vi "PPL Version Pre-Build Action.vi"(6 "Top Level/Always Included VIs":path[](array[path]), 7 "Main Destination Path":path, 9 "Target Name":string, 10 "Build Specification Name":string, 11 "Project Path":path) -> (0 "error out":errorcluster)   [LabVIEW 2023]
panel:
  in  "error in (no error)":errorcluster
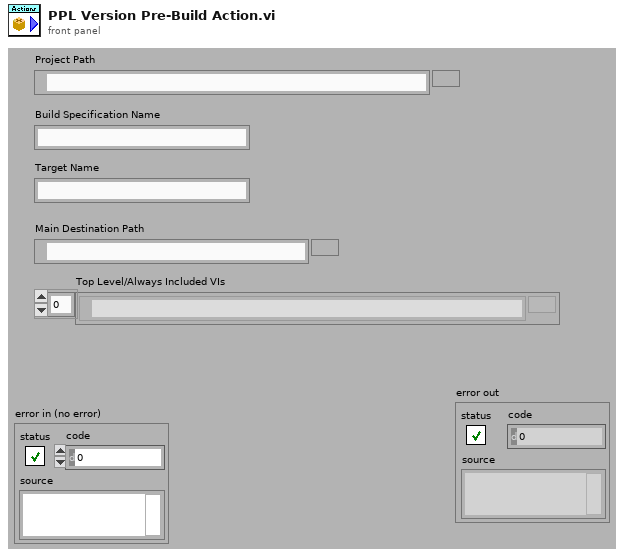
[diagram p1: front panel]
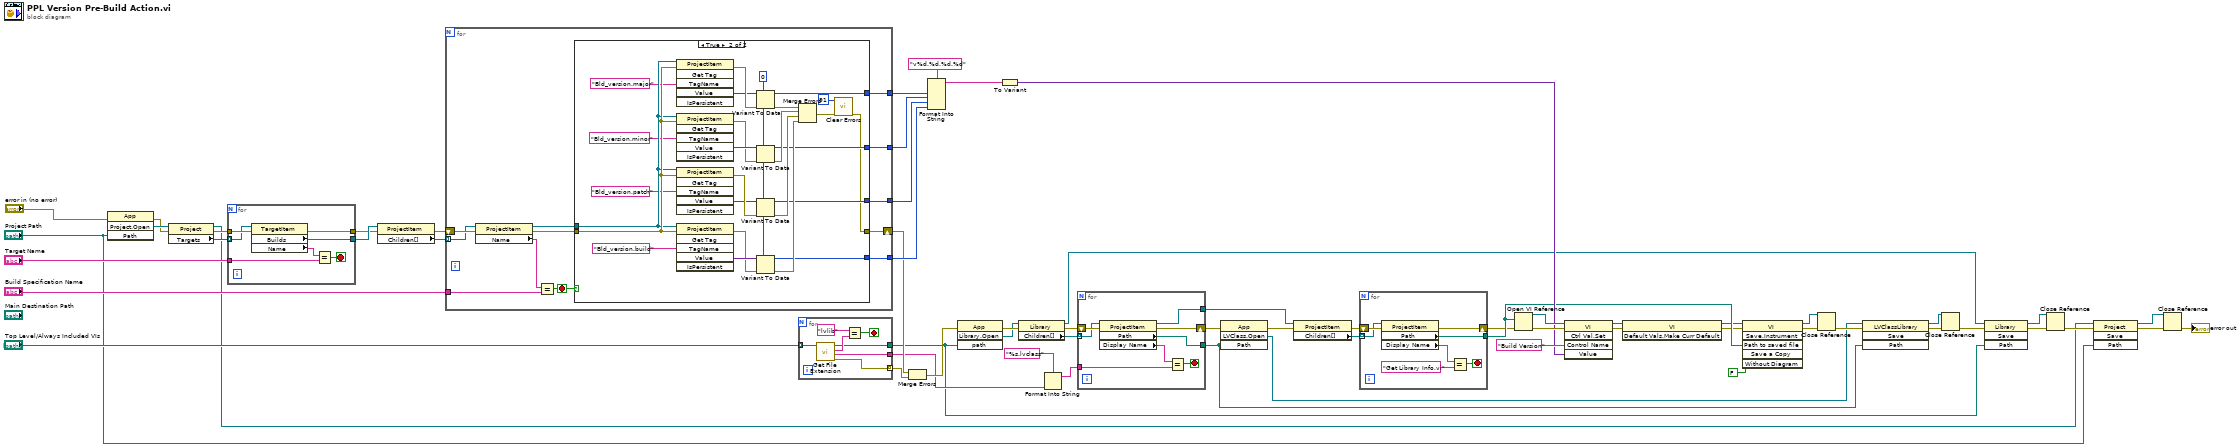
[diagram p0: block diagram]
diagram:
  n1 = invoke class="App" method="Project.Open"(error in="error in (no error)", "Path"="Project Path") -> (error out=w59:errorcluster, "Project:Open"=w62:refnum<vi>)  [unwired: 2 in, 2 out]
  n2 = property class="Project"(reference=w62, error in=w59) -> (reference out=w14:refnum<vi>, error out=w58:errorcluster, "Targets"=w60:refnum<vi>[])
  n3 = for {
    tunnel: w60 -> [w68] mode=indexing
    tunnel: w58 -> [w69]
    tunnel: "Target Name" -> [w67]
    tunnel: [w65] -> w56
    tunnel: [w63] -> w57
    stop <- w66 stop-if-true
    n4 = property class="TargetItem"(reference=w68, error in=w69) -> (error out=w65:errorcluster, "Builds"=w63:refnum<vi>, "Name"=w64:string)  [unwired: 1 out]
    n5 = Equal?(x=w64, y=w67) -> (x = y?=w66:bool)
  }
  n6 = property class="ProjectItem"(reference=w57, error in=w56) -> (error out=w55:errorcluster, "Children[]"=w54:refnum<vi>[])  [unwired: 1 out]
  n7 = for {
    tunnel: "Build Specification Name" -> [w80]
    shift-right: [w79] -> w45
    shift-left: w55 -> [w78]
    tunnel: w54 -> [w77] mode=indexing
    tunnel: [w74] -> w52
    tunnel: [w72] -> w51
    tunnel: [w71] -> w50
    tunnel: [w70] -> w49
    stop <- w73 stop-if-true
    n8 = property class="ProjectItem"(reference=w77) -> (reference out=w75:refnum<vi>, "Name"=w76:string)  [unwired: 1 in, 1 out]
    n9 = Equal?(x=w76, y=w80) -> (x = y?=w73:bool)
    n10 = case shown="True" w73 {
      tunnel: w78 -> [w81 w107]
      tunnel: w75 -> [_ w106]
      tunnel: [w81 w83] -> w79
      tunnel: [_ w89] -> w74
      tunnel: [_ w88] -> w72
      tunnel: [_ w87] -> w71
      tunnel: [_ w86] -> w70
      frame False {
      }
      frame True {
        w93 = u32 0
        n11 = invoke class="ProjectItem" method="Get Tag"(reference=w106, error in=w107, "TagName"="Bld_version.major") -> (error out=w101:errorcluster, "Value"=w100:variant)  [unwired: 3 in, 4 out]
        n12 = invoke class="ProjectItem" method="Get Tag"(reference=w106, error in=w107, "TagName"="Bld_version.minor") -> (error out=w98:errorcluster, "Value"=w99:variant)  [unwired: 3 in, 4 out]
        n13 = invoke class="ProjectItem" method="Get Tag"(reference=w106, error in=w107, "TagName"="Bld_version.patch") -> (error out=w95:errorcluster, "Value"=w94:variant)  [unwired: 3 in, 4 out]
        n14 = invoke class="ProjectItem" method="Get Tag"(reference=w106, error in=w107, "TagName"="Bld_version.build") -> (error out=w96:errorcluster, "Value"=w97:variant)  [unwired: 3 in, 4 out]
        n15 = Variant To Data(error in=w101, type=w93, Variant=w100) -> (data=w89:u32, error out=w85:errorcluster)
        n16 = Variant To Data(error in=w98, type=w93, Variant=w99) -> (data=w88:u32, error out=w92:errorcluster)
        n17 = Variant To Data(error in=w95, type=w93, Variant=w94) -> (data=w87:u32, error out=w91:errorcluster)
        n18 = Variant To Data(error in=w96, type=w93, Variant=w97) -> (data=w86:u32, error out=w90:errorcluster)
        n19 = Merge Errors(w85, w92, w91, w90) -> (w84:errorcluster)
        n20 = call <vilib>:"Clear Errors.vi"("error in (no error)"=w84, "specific error code to clear (0: all)"=91) -> ("error out"=w83:errorcluster)  [unwired: 4 in, 1 out]
      }
    }
  }
  n21 = for {
    tunnel: "Top Level/Always Included VIs" -> [w114] mode=indexing
    tunnel: [w110] -> w18
    tunnel: [w109] -> w44 mode=indexing
    tunnel: [w108] -> w30
    stop <- w111 stop-if-true
    n22 = call <vilib>:"Get File Extension.vi"("file"=w114) -> ("error out"=w109:errorcluster, "filename without extension"=w108:string, "lowercase file extension"=w113:string, "dup file"=w110:path)  [unwired: 6 in, 1 out]
    n23 = Equal?(x="lvlib", y=w113) -> (x = y?=w111:bool)
  }
  n24 = Merge Errors(w45, w44) -> (w36:errorcluster)
  n25 = Format Into String(format string="v%d.%d.%d.%d", w52, w51, w50, w49) -> (resulting string=w40:string)  [unwired: 2 in, 1 out]
  n26 = invoke class="App" method="Library.Open"(error in=w36, "path"=w18) -> (error out=w35:errorcluster, "Open Library"=w34:refnum<vi>)  [unwired: 2 in, 2 out]
  n27 = To Variant(anything=w40) -> (Variant=w39:variant)
  n28 = property class="Library"(reference=w34, error in=w35) -> (reference out=w19:refnum<vi>, error out=w32:errorcluster, "Children[]"=w33:refnum<vi>[])
  n29 = Format Into String(format string="%s.lvclass", w30) -> (resulting string=w29:string)  [unwired: 2 in, 1 out]
  n30 = for {
    tunnel: w33 -> [w121] mode=indexing
    shift-right: [w118] -> w9
    shift-left: w32 -> [w122]
    tunnel: w29 -> [w120]
    tunnel: [w117] -> w7
    tunnel: [w115] -> w4
    stop <- w119 stop-if-true
    n31 = property class="ProjectItem"(reference=w121, error in=w122) -> (reference out=w117:refnum<vi>, error out=w118:errorcluster, "Path"=w115:path, "Display Name"=w116:string)
    n32 = Equal?(x=w116, y=w120) -> (x = y?=w119:bool)
  }
  n33 = invoke class="App" method="LVClass.Open"(error in=w9, "Path"=w4) -> (error out=w8:errorcluster, "LVClass.Open"=w5:refnum<vi>)  [unwired: 2 in, 2 out]
  n34 = property class="ProjectItem"(reference=w7, error in=w8) -> (error out=w28:errorcluster, "Children[]"=w27:refnum<vi>[])  [unwired: 1 out]
  n35 = for {
    tunnel: w27 -> [w128] mode=indexing
    shift-right: [w126] -> w25
    shift-left: w28 -> [w129]
    tunnel: [w123] -> w26
    stop <- w127 stop-if-true
    n36 = property class="ProjectItem"(reference=w128, error in=w129) -> (error out=w126:errorcluster, "Path"=w123:path, "Display Name"=w124:string)  [unwired: 1 out]
    n37 = Equal?(x=w124, y="Get Library Info.vi") -> (x = y?=w127:bool)
  }
  n38 = Open VI Reference(vi path=w26, error in (no error)=w25) -> (vi reference=w42:refnum<vi>, error out=w43:errorcluster)  [unwired: 4 in]
  n39 = invoke class="VI" method="Ctrl Val.Set"(reference=w42, error in=w43, "Control Name"="Build Version", "Value"=w39) -> (reference out=w23:refnum<vi>, error out=w24:errorcluster)  [unwired: 1 in, 3 out]
  n40 = invoke class="VI" method="Default Vals.Make Curr Default"(reference=w23, error in=w24) -> (reference out=w21:refnum<vi>, error out=w22:errorcluster)  [unwired: 1 in, 1 out]
  n41 = invoke class="VI" method="Save.Instrument"(reference=w21, error in=w22, "Path to saved file"=w26, "Without Diagram"=FALSE) -> (reference out=w37:refnum<vi>, error out=w38:errorcluster)  [unwired: 2 in, 4 out]
  n42 = Close Reference(reference=w37, error in (no error)=w38) -> (error out=w6:errorcluster)
  n43 = invoke class="LVClassLibrary" method="Save"(reference=w5, error in=w6, "Path"=w4) -> (reference out=w2:refnum<vi>, error out=w3:errorcluster)  [unwired: 1 in, 2 out]
  n44 = Close Reference(reference=w2, error in (no error)=w3) -> (error out=w1:errorcluster)
  n45 = invoke class="Library" method="Save"(reference=w19, error in=w1, "Path"=w18) -> (reference out=w17:refnum<vi>, error out=w16:errorcluster)  [unwired: 1 in, 2 out]
  n46 = Close Reference(reference=w17, error in (no error)=w16) -> (error out=w15:errorcluster)
  n47 = invoke class="Project" method="Save"(reference=w14, error in=w15, "Path"="Project Path") -> (reference out=w11:refnum<vi>, error out=w12:errorcluster)  [unwired: 1 in, 2 out]
  n48 = Close Reference(reference=w11, error in (no error)=w12) -> (error out=→"error out":errorcluster)
